vi "Changing CANCoder Zeros.vi"() -> ()   [LabVIEW 2020]
uses:
  <vilib>/Rock Robotics/WPI/ThirdParty/Phoenix-LabVIEW/CANCoder/Get/CTRE_Phoenix_CANcoder_GetSensorData.vi
  <vilib>/Rock Robotics/WPI/ThirdParty/Phoenix-LabVIEW/CANCoder/Controls/CTRE_Phoenix_CANcoder_DeviceRef.ctl
panel:
  out "cancoder \"zeros\"":cluster{"10":dbl, "12":dbl, "11":dbl, "9":dbl}={"10"=-45.0, "12"=-63.6328, "11"=-157.061, "9"=19.7754}
  in  "Input Cancoders":T2
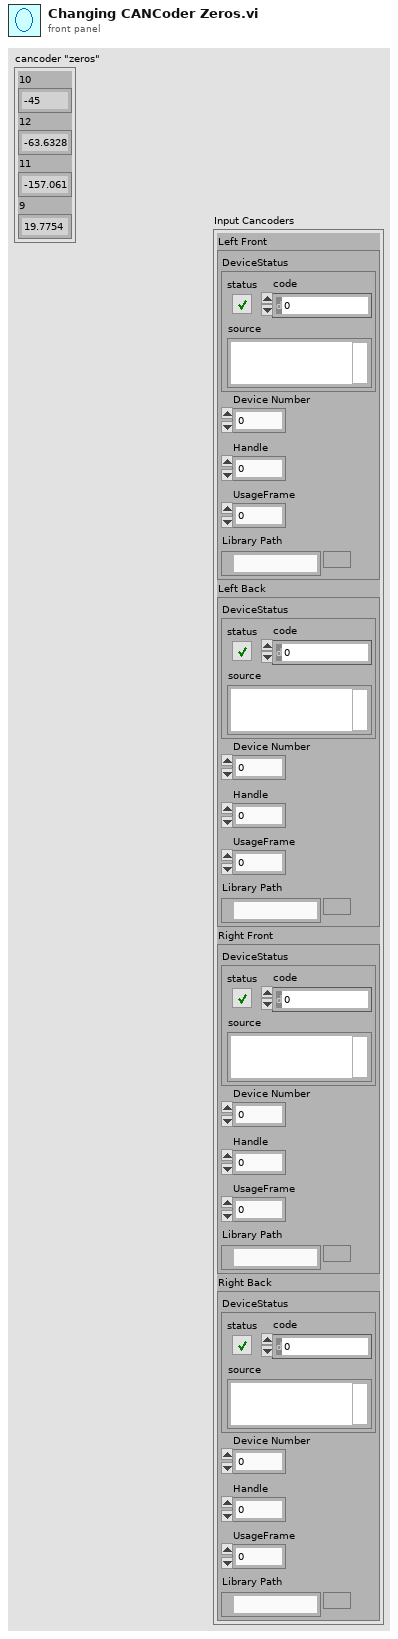
[diagram p1: front panel]
types:
  T1 = typedef "CTRE_Phoenix_CANcoder_DeviceRef.ctl" = cluster{"DeviceStatus":errorcluster, "Device Number":u8, "Handle":u64, "UsageFrame":u32, "Library Path":path}
  T2 = cluster{"Left Front":T1, "Left Back":T1, "Right Front":T1, "Right Back":T1}
  T3 = cluster{"Absolute Position":dbl, "Absolute Position":dbl, "Absolute Position":dbl, "Absolute Position":dbl}
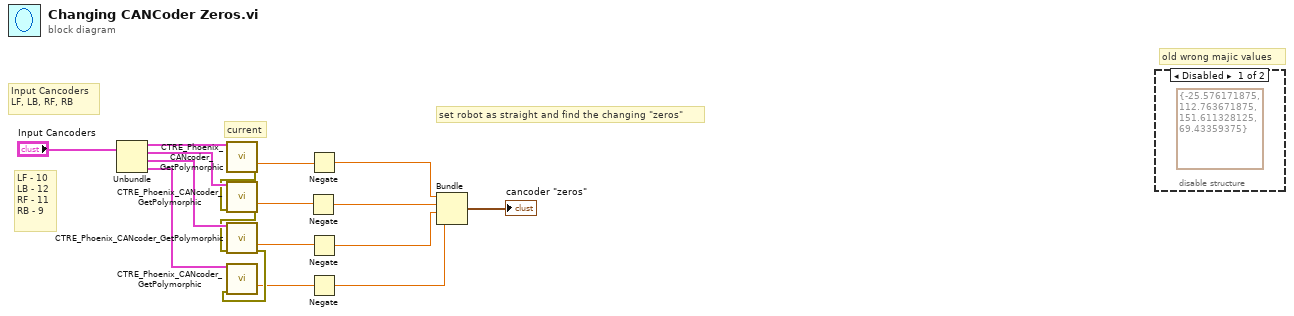
[diagram p0: block diagram]
diagram:
  # "set robot as straight and find the changing \"zeros\""
  # "current"
  # "old wrong majic values"
  # "LF - 10 \nLB - 12\nRF - 11\nRB - 9"
  # "Input Cancoders\nLF, LB, RF, RB"
  n1 = Unbundle("Input Cancoders") -> ("Left Front"=w16:T1, "Left Back"=w15:T1, "Right Front"=w14:T1, "Right Back"=w13:T1)
  n2 = call-poly <vilib>:"CTRE_Phoenix_CANcoder_GetPolymorphic.vi"("CTRE_CANcoder_DeviceRef"=w16) -> ("Absolute Position"=w9:dbl, "error out"=w12:errorcluster)  [unwired: 10 in, 3 out]
  n3 = call-poly <vilib>:"CTRE_Phoenix_CANcoder_GetPolymorphic.vi"("CTRE_CANcoder_DeviceRef"=w15, "error in"=w12) -> ("Absolute Position"=w8:dbl, "error out"=w11:errorcluster)  [unwired: 9 in, 3 out]
  n4 = call-poly <vilib>:"CTRE_Phoenix_CANcoder_GetPolymorphic.vi"("CTRE_CANcoder_DeviceRef"=w14, "error in"=w11) -> ("Absolute Position"=w7:dbl, "error out"=w10:errorcluster)  [unwired: 9 in, 3 out]
  n5 = call-poly <vilib>:"CTRE_Phoenix_CANcoder_GetPolymorphic.vi"("CTRE_CANcoder_DeviceRef"=w13, "error in"=w10) -> ("Absolute Position"=w6:dbl)  [unwired: 9 in, 4 out]
  n6 = Negate(x=w8) -> (-x=w4:dbl)
  n7 = Negate(x=w9) -> (-x=w5:dbl)
  n8 = Negate(x=w7) -> (-x=w3:dbl)
  n9 = Negate(x=w6) -> (-x=w2:dbl)
  n10 = Bundle(w5, w4, w3, w2) -> (→"cancoder \"zeros\"":cluster{dbl, dbl, dbl, dbl})  [unwired: 1 in]
  n11 = disable-structure shown="Disabled" {
    frame Disabled {
      (unwired) T3 {"Absolute Position"=-25.576171875, "Absolute Position"=112.763671875, "Absolute Position"=151.611328125, "Absolute Position"=69.43359375} ("Absolute Positions")
    }
    frame Enabled {
    }
  }
